vi "Open.vi"(8 "error in (no error)":errorcluster, 10 "address":string, 11 "Inst.Magneto in":refnum<class "Inst.Magneto.lvclass">) -> (0 "error out":errorcluster, 3 "Inst.Magneto out":refnum<class "Inst.Magneto.lvclass">)   [LabVIEW 2019, in "Inst.Magneto.lvclass"]
uses:
  Inst.Magneto.lvclass
  C:/Program Files (x86)/National Instruments/LabVIEW 2019/user.lib/LevyLab/Instrument Framework/SMOs/Instrument/Instrument.lvclass
  <userlib>/Levylab/Instrument Framework/Instrument Types/VSource/Instrument.VSource.lvclass
  <userlib>/LevyLab/Instrument Framework/SMOs/Instrument/Instrument.lvclass
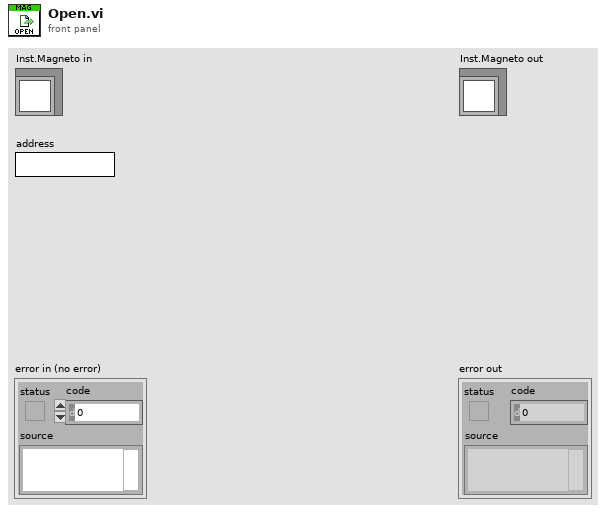
[diagram p1: front panel]
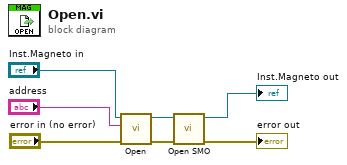
[diagram p0: block diagram]
diagram:
  n1 = call-parent "Open.vi"("error in (no error)"="error in (no error)", "address"="address", "Instrument in"="Inst.Magneto in") -> ("error out"=w4:errorcluster, "Instrument out"=w3:refnum<class "Inst.Magneto.lvclass">)  [unwired: 7 in]
  n2 = call <userlib>:"Open SMO.vi"("error in (no error)"=w4, "Instrument in"=w3) -> ("error out"=→"error out":errorcluster, "Instrument out"=→"Inst.Magneto out":refnum<class "Inst.Magneto.lvclass">)  [unwired: 8 in]
